vi "increment Modbus address.vi"(0 "available addresses":T1(array[cluster]), 5 "modbus type":T2, 7 "data type":T3) -> (4 "available addresses out":T1(array[cluster]), 6 "starting address":u16, 8 "subindex (bool)":i32)   [LabVIEW 2013, in "Modbus Slave configuration.lvclass"]
uses:
  Modbus Slave configuration.lvclass
  <vilib>/NI/Tag Bus/tag/Data Type.ctl
  <vilib>/NI/Tag Bus/tag/tag descriptor.lvclass
  module channel/data bank type.ctl
  module channel/Modbus Module Channel.lvclass
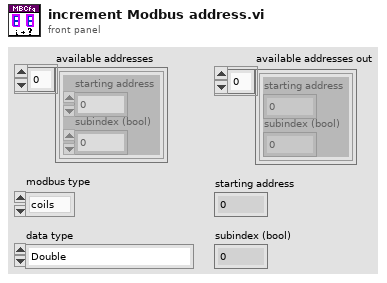
[diagram p1: front panel]
types:
  T1 = cluster{"starting address":u16, "subindex (bool)":i32}[]
  T2 = typedef "Modbus Module Channel.lvclass/data bank type.ctl" = enum16{"coils", "discrete inputs", "input registers", "holding registers"}
  T3 = typedef "tag bus.lvlib/tag descriptor.lvclass/Data Type.ctl" = enum16{"Double", "Single", "I64", "I32", "I16", "I8", "U64", "U32", "U16", "U8", "Boolean", "String", "Array of Double", "Array of Single", "Array of I64", "Array of I32", "Array of I16", "Array of I8", "Array of U64", "Array of U32", "Array of U16", "Array of U8", "Array of Boolean", "Array of String"}
  T4 = cluster{"starting address":u16, "subindex (bool)":i32}
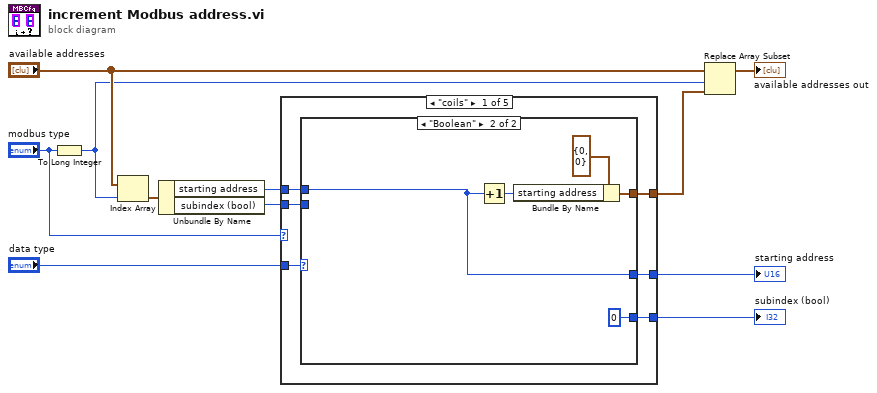
[diagram p0: block diagram]
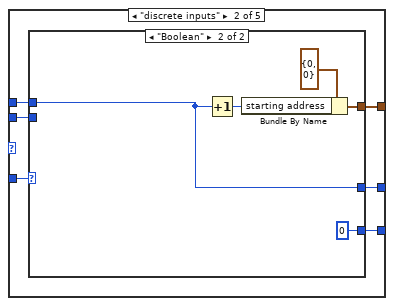
[diagram p3: hidden frame]
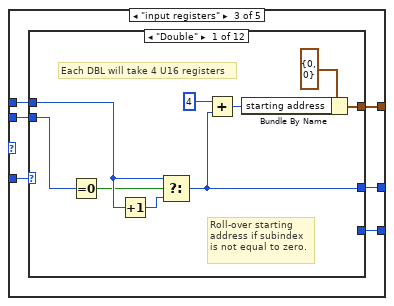
[diagram p5: hidden frame]
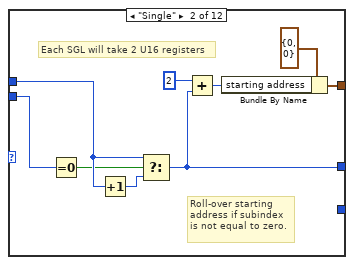
[diagram p6: hidden frame]
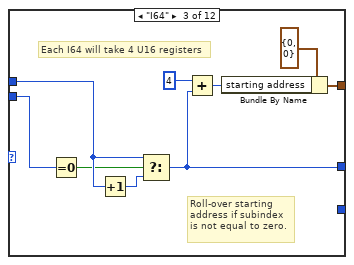
[diagram p7: hidden frame]
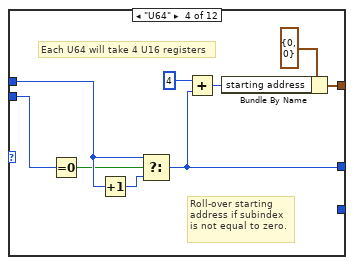
[diagram p8: hidden frame]
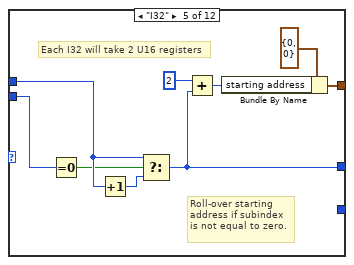
[diagram p9: hidden frame]
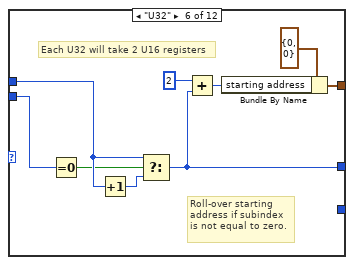
[diagram p10: hidden frame]
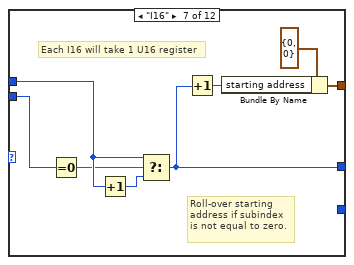
[diagram p11: hidden frame]
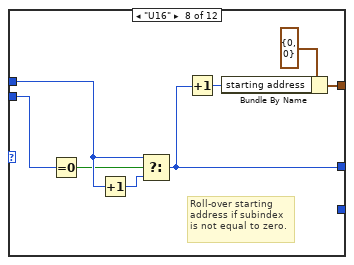
[diagram p12: hidden frame]
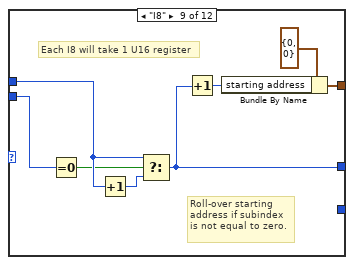
[diagram p13: hidden frame]
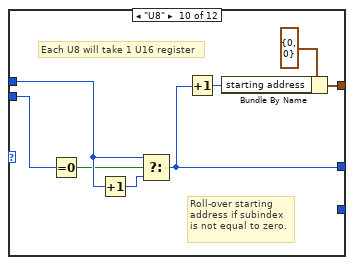
[diagram p14: hidden frame]
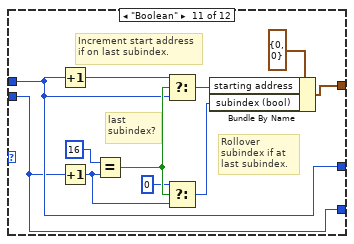
[diagram p15: hidden frame]
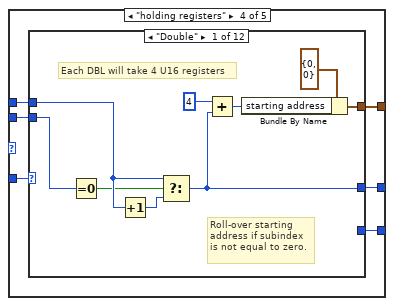
[diagram p17: hidden frame]
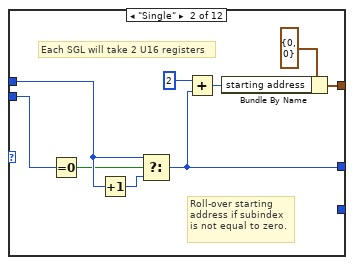
[diagram p18: hidden frame]
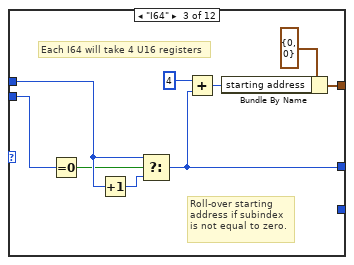
[diagram p19: hidden frame]
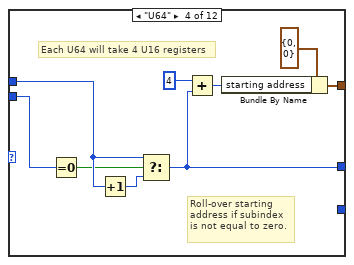
[diagram p20: hidden frame]
diagram:
  n1 = To Long Integer(number="modbus type") -> (32bit integer=w8:i32)
  n2 = Index Array(array="available addresses", index=w8) -> (element=w10:T4)
  n3 = Unbundle By Name(w10) -> ("starting address"=w4:u16, "subindex (bool)"=w7:i32)
  n4 = case shown="\"coils\"" "modbus type" {
    tunnel: "data type" -> [w17 w28 w39 w142 _]
    tunnel: w7 -> [w16 w27 w38 w141 _]
    tunnel: [w15 w26 w37 w140 _] -> w5
    tunnel: w4 -> [w14 w25 w36 w139 _]
    tunnel: [w13 w24 w35 w138 _] -> w3
    tunnel: [w12 w23 w34 w137 _] -> w2
    frame "coils" {
      n5 = case shown="\"Boolean\"" w17 {
        tunnel: w16 -> [_ _]
        tunnel: w14 -> [_ w18]
        tunnel: [_ w21] -> w15
        tunnel: [_ w18] -> w13
        tunnel: [_ 0 ("subindex (bool)")] -> w12
        frame Default {
        }
        frame "Boolean" {
          n6 = Increment(x=w18) -> (x+1=w20:u16)
          n7 = Bundle By Name(cluster=T4 {"starting address"=0, "subindex (bool)"=0} ("element"), "starting address"=w20) -> (w21:T4)
        }
      }
    }
    frame "discrete inputs" {
      n8 = case shown="\"Boolean\"" w28 {
        tunnel: w27 -> [_ _]
        tunnel: w25 -> [_ w29]
        tunnel: [_ w32] -> w26
        tunnel: [_ w29] -> w24
        tunnel: [_ 0 ("subindex (bool)")] -> w23
        frame Default {
        }
        frame "Boolean" {
          n9 = Increment(x=w29) -> (x+1=w31:u16)
          n10 = Bundle By Name(cluster=T4 {"starting address"=0, "subindex (bool)"=0} ("element"), "starting address"=w31) -> (w32:T4)
        }
      }
    }
    frame "input registers" {
      n11 = case shown="\"Double\"" w39 {
        tunnel: w38 -> [w45 w54 w63 w72 w81 w90 w99 w107 w115 w123 w126 _]
        tunnel: w36 -> [w44 w53 w62 w71 w80 w89 w98 w106 w114 w122 w127 _]
        tunnel: [w47 w56 w65 w74 w83 w92 w100 w108 w116 w124 w135 _] -> w37
        tunnel: [w41 w50 w59 w68 w77 w86 w95 w103 w111 w119 w127 _] -> w35
        tunnel: [_ _ _ _ _ _ _ _ _ _ w126 _] -> w34
        frame "Double" {
          # "Each DBL will take 4 U16 registers"
          # "Roll-over starting\naddress if subindex\nis not equal to zero."
          n12 = Equal To 0?(x=w45) -> (x = 0?=w42:bool)
          n13 = Increment(x=w44) -> (x+1=w43:u16)
          n14 = Select(t=w44, s=w42, f=w43) -> (s? t:f=w41:u16)
          n15 = Add(x=u16 4, y=w41) -> (x+y=w40:u16)
          n16 = Bundle By Name(cluster=T4 {"starting address"=0, "subindex (bool)"=0} ("element"), "starting address"=w40) -> (w47:T4)
        }
        frame "Single" {
          # "Each SGL will take 2 U16 registers"
          # "Roll-over starting\naddress if subindex\nis not equal to zero."
          n17 = Equal To 0?(x=w54) -> (x = 0?=w51:bool)
          n18 = Increment(x=w53) -> (x+1=w52:u16)
          n19 = Select(t=w53, s=w51, f=w52) -> (s? t:f=w50:u16)
          n20 = Add(x=u16 2, y=w50) -> (x+y=w49:u16)
          n21 = Bundle By Name(cluster=T4 {"starting address"=0, "subindex (bool)"=0} ("element"), "starting address"=w49) -> (w56:T4)
        }
        frame "I64" {
          # "Each I64 will take 4 U16 registers"
          # "Roll-over starting\naddress if subindex\nis not equal to zero."
          n22 = Equal To 0?(x=w63) -> (x = 0?=w60:bool)
          n23 = Increment(x=w62) -> (x+1=w61:u16)
          n24 = Select(t=w62, s=w60, f=w61) -> (s? t:f=w59:u16)
          n25 = Add(x=u16 4, y=w59) -> (x+y=w58:u16)
          n26 = Bundle By Name(cluster=T4 {"starting address"=0, "subindex (bool)"=0} ("element"), "starting address"=w58) -> (w65:T4)
        }
        frame "U64" {
          # "Each U64 will take 4 U16 registers"
          # "Roll-over starting\naddress if subindex\nis not equal to zero."
          n27 = Equal To 0?(x=w72) -> (x = 0?=w69:bool)
          n28 = Increment(x=w71) -> (x+1=w70:u16)
          n29 = Select(t=w71, s=w69, f=w70) -> (s? t:f=w68:u16)
          n30 = Add(x=u16 4, y=w68) -> (x+y=w67:u16)
          n31 = Bundle By Name(cluster=T4 {"starting address"=0, "subindex (bool)"=0} ("element"), "starting address"=w67) -> (w74:T4)
        }
        frame "I32" {
          # "Each I32 will take 2 U16 registers"
          # "Roll-over starting\naddress if subindex\nis not equal to zero."
          n32 = Equal To 0?(x=w81) -> (x = 0?=w78:bool)
          n33 = Increment(x=w80) -> (x+1=w79:u16)
          n34 = Select(t=w80, s=w78, f=w79) -> (s? t:f=w77:u16)
          n35 = Add(x=u16 2, y=w77) -> (x+y=w76:u16)
          n36 = Bundle By Name(cluster=T4 {"starting address"=0, "subindex (bool)"=0} ("element"), "starting address"=w76) -> (w83:T4)
        }
        frame "U32" {
          # "Each U32 will take 2 U16 registers"
          # "Roll-over starting\naddress if subindex\nis not equal to zero."
          n37 = Equal To 0?(x=w90) -> (x = 0?=w87:bool)
          n38 = Increment(x=w89) -> (x+1=w88:u16)
          n39 = Select(t=w89, s=w87, f=w88) -> (s? t:f=w86:u16)
          n40 = Add(x=u16 2, y=w86) -> (x+y=w85:u16)
          n41 = Bundle By Name(cluster=T4 {"starting address"=0, "subindex (bool)"=0} ("element"), "starting address"=w85) -> (w92:T4)
        }
        frame "I16" {
          # "Each I16 will take 1 U16 register"
          # "Roll-over starting\naddress if subindex\nis not equal to zero."
          n42 = Equal To 0?(x=w99) -> (x = 0?=w96:bool)
          n43 = Increment(x=w98) -> (x+1=w97:u16)
          n44 = Select(t=w98, s=w96, f=w97) -> (s? t:f=w95:u16)
          n45 = Increment(x=w95) -> (x+1=w94:u16)
          n46 = Bundle By Name(cluster=T4 {"starting address"=0, "subindex (bool)"=0} ("element"), "starting address"=w94) -> (w100:T4)
        }
        frame "U16" {
          # "Roll-over starting\naddress if subindex\nis not equal to zero."
          n47 = Equal To 0?(x=w107) -> (x = 0?=w104:bool)
          n48 = Increment(x=w106) -> (x+1=w105:u16)
          n49 = Select(t=w106, s=w104, f=w105) -> (s? t:f=w103:u16)
          n50 = Increment(x=w103) -> (x+1=w102:u16)
          n51 = Bundle By Name(cluster=T4 {"starting address"=0, "subindex (bool)"=0} ("element"), "starting address"=w102) -> (w108:T4)
        }
        frame "I8" {
          # "Each I8 will take 1 U16 register"
          # "Roll-over starting\naddress if subindex\nis not equal to zero."
          n52 = Equal To 0?(x=w115) -> (x = 0?=w112:bool)
          n53 = Increment(x=w114) -> (x+1=w113:u16)
          n54 = Select(t=w114, s=w112, f=w113) -> (s? t:f=w111:u16)
          n55 = Increment(x=w111) -> (x+1=w110:u16)
          n56 = Bundle By Name(cluster=T4 {"starting address"=0, "subindex (bool)"=0} ("element"), "starting address"=w110) -> (w116:T4)
        }
        frame "U8" {
          # "Each U8 will take 1 U16 register"
          # "Roll-over starting\naddress if subindex\nis not equal to zero."
          n57 = Equal To 0?(x=w123) -> (x = 0?=w120:bool)
          n58 = Increment(x=w122) -> (x+1=w121:u16)
          n59 = Select(t=w122, s=w120, f=w121) -> (s? t:f=w119:u16)
          n60 = Increment(x=w119) -> (x+1=w118:u16)
          n61 = Bundle By Name(cluster=T4 {"starting address"=0, "subindex (bool)"=0} ("element"), "starting address"=w118) -> (w124:T4)
        }
        frame "Boolean" {
          # "Increment start address\nif on last subindex."
          # "Rollover subindex if at last subindex."
          # "last\nsubindex?"
          n62 = Increment(x=w127) -> (x+1=w129:u16)
          n63 = Increment(x=w126) -> (x+1=w128:i32)
          n64 = Equal?(x=16, y=w128) -> (x = y?=w133:bool)
          n65 = Select(t=w129, s=w133, f=w127) -> (s? t:f=w131:u16)
          n66 = Select(t=0, s=w133, f=w128) -> (s? t:f=w130:i32)
          n67 = Bundle By Name(cluster=T4 {"starting address"=0, "subindex (bool)"=0} ("element"), "starting address"=w131, "subindex (bool)"=w130) -> (w135:T4)
        }
        frame Default {
        }
      }
    }
    frame "holding registers" {
      n68 = case shown="\"Double\"" w142 {
        tunnel: w141 -> [w148 w157 w166 w175 w184 w193 w202 w210 w218 w226 w229 _]
        tunnel: w139 -> [w147 w156 w165 w174 w183 w192 w201 w209 w217 w225 w230 _]
        tunnel: [w150 w159 w168 w177 w186 w195 w203 w211 w219 w227 w238 _] -> w140
        tunnel: [w144 w153 w162 w171 w180 w189 w198 w206 w214 w222 w230 _] -> w138
        tunnel: [_ _ _ _ _ _ _ _ _ _ w229 _] -> w137
        frame "Double" {
          # "Each DBL will take 4 U16 registers"
          # "Roll-over starting\naddress if subindex\nis not equal to zero."
          n69 = Equal To 0?(x=w148) -> (x = 0?=w145:bool)
          n70 = Increment(x=w147) -> (x+1=w146:u16)
          n71 = Select(t=w147, s=w145, f=w146) -> (s? t:f=w144:u16)
          n72 = Add(x=u16 4, y=w144) -> (x+y=w143:u16)
          n73 = Bundle By Name(cluster=T4 {"starting address"=0, "subindex (bool)"=0} ("element"), "starting address"=w143) -> (w150:T4)
        }
        frame "Single" {
          # "Each SGL will take 2 U16 registers"
          # "Roll-over starting\naddress if subindex\nis not equal to zero."
          n74 = Equal To 0?(x=w157) -> (x = 0?=w154:bool)
          n75 = Increment(x=w156) -> (x+1=w155:u16)
          n76 = Select(t=w156, s=w154, f=w155) -> (s? t:f=w153:u16)
          n77 = Add(x=u16 2, y=w153) -> (x+y=w152:u16)
          n78 = Bundle By Name(cluster=T4 {"starting address"=0, "subindex (bool)"=0} ("element"), "starting address"=w152) -> (w159:T4)
        }
        frame "I64" {
          # "Each I64 will take 4 U16 registers"
          # "Roll-over starting\naddress if subindex\nis not equal to zero."
          n79 = Equal To 0?(x=w166) -> (x = 0?=w163:bool)
          n80 = Increment(x=w165) -> (x+1=w164:u16)
          n81 = Select(t=w165, s=w163, f=w164) -> (s? t:f=w162:u16)
          n82 = Add(x=u16 4, y=w162) -> (x+y=w161:u16)
          n83 = Bundle By Name(cluster=T4 {"starting address"=0, "subindex (bool)"=0} ("element"), "starting address"=w161) -> (w168:T4)
        }
        frame "U64" {
          # "Each U64 will take 4 U16 registers"
          # "Roll-over starting\naddress if subindex\nis not equal to zero."
          n84 = Equal To 0?(x=w175) -> (x = 0?=w172:bool)
          n85 = Increment(x=w174) -> (x+1=w173:u16)
          n86 = Select(t=w174, s=w172, f=w173) -> (s? t:f=w171:u16)
          n87 = Add(x=u16 4, y=w171) -> (x+y=w170:u16)
          n88 = Bundle By Name(cluster=T4 {"starting address"=0, "subindex (bool)"=0} ("element"), "starting address"=w170) -> (w177:T4)
        }
        frame "I32" {
          # "Each I32 will take 2 U16 registers"
          # "Roll-over starting\naddress if subindex\nis not equal to zero."
          n89 = Equal To 0?(x=w184) -> (x = 0?=w181:bool)
          n90 = Increment(x=w183) -> (x+1=w182:u16)
          n91 = Select(t=w183, s=w181, f=w182) -> (s? t:f=w180:u16)
          n92 = Add(x=u16 2, y=w180) -> (x+y=w179:u16)
          n93 = Bundle By Name(cluster=T4 {"starting address"=0, "subindex (bool)"=0} ("element"), "starting address"=w179) -> (w186:T4)
        }
        frame "U32" {
          # "Each U32 will take 2 U16 registers"
          # "Roll-over starting\naddress if subindex\nis not equal to zero."
          n94 = Equal To 0?(x=w193) -> (x = 0?=w190:bool)
          n95 = Increment(x=w192) -> (x+1=w191:u16)
          n96 = Select(t=w192, s=w190, f=w191) -> (s? t:f=w189:u16)
          n97 = Add(x=u16 2, y=w189) -> (x+y=w188:u16)
          n98 = Bundle By Name(cluster=T4 {"starting address"=0, "subindex (bool)"=0} ("element"), "starting address"=w188) -> (w195:T4)
        }
        frame "I16" {
          # "Each I16 will take 1 U16 register"
          # "Roll-over starting\naddress if subindex\nis not equal to zero."
          n99 = Equal To 0?(x=w202) -> (x = 0?=w199:bool)
          n100 = Increment(x=w201) -> (x+1=w200:u16)
          n101 = Select(t=w201, s=w199, f=w200) -> (s? t:f=w198:u16)
          n102 = Increment(x=w198) -> (x+1=w197:u16)
          n103 = Bundle By Name(cluster=T4 {"starting address"=0, "subindex (bool)"=0} ("element"), "starting address"=w197) -> (w203:T4)
        }
        frame "U16" {
          # "Roll-over starting\naddress if subindex\nis not equal to zero."
          n104 = Equal To 0?(x=w210) -> (x = 0?=w207:bool)
          n105 = Increment(x=w209) -> (x+1=w208:u16)
          n106 = Select(t=w209, s=w207, f=w208) -> (s? t:f=w206:u16)
          n107 = Increment(x=w206) -> (x+1=w205:u16)
          n108 = Bundle By Name(cluster=T4 {"starting address"=0, "subindex (bool)"=0} ("element"), "starting address"=w205) -> (w211:T4)
        }
        frame "I8" {
          # "Each I8 will take 1 U16 register"
          # "Roll-over starting\naddress if subindex\nis not equal to zero."
          n109 = Equal To 0?(x=w218) -> (x = 0?=w215:bool)
          n110 = Increment(x=w217) -> (x+1=w216:u16)
          n111 = Select(t=w217, s=w215, f=w216) -> (s? t:f=w214:u16)
          n112 = Increment(x=w214) -> (x+1=w213:u16)
          n113 = Bundle By Name(cluster=T4 {"starting address"=0, "subindex (bool)"=0} ("element"), "starting address"=w213) -> (w219:T4)
        }
        frame "U8" {
          # "Each U8 will take 1 U16 register"
          # "Roll-over starting\naddress if subindex\nis not equal to zero."
          n114 = Equal To 0?(x=w226) -> (x = 0?=w223:bool)
          n115 = Increment(x=w225) -> (x+1=w224:u16)
          n116 = Select(t=w225, s=w223, f=w224) -> (s? t:f=w222:u16)
          n117 = Increment(x=w222) -> (x+1=w221:u16)
          n118 = Bundle By Name(cluster=T4 {"starting address"=0, "subindex (bool)"=0} ("element"), "starting address"=w221) -> (w227:T4)
        }
        frame "Boolean" {
          # "Increment start address\nif on last subindex."
          # "Rollover subindex if at last subindex."
          # "last\nsubindex?"
          n119 = Increment(x=w230) -> (x+1=w232:u16)
          n120 = Increment(x=w229) -> (x+1=w231:i32)
          n121 = Equal?(x=16, y=w231) -> (x = y?=w236:bool)
          n122 = Select(t=w232, s=w236, f=w230) -> (s? t:f=w234:u16)
          n123 = Select(t=0, s=w236, f=w231) -> (s? t:f=w233:i32)
          n124 = Bundle By Name(cluster=T4 {"starting address"=0, "subindex (bool)"=0} ("element"), "starting address"=w234, "subindex (bool)"=w233) -> (w238:T4)
        }
        frame Default {
        }
      }
    }
    frame Default {
    }
  }
  "subindex (bool)" <- w2
  "starting address" <- w3
  n125 = Replace Array Subset(array="available addresses", new element=w5, index=w8) -> (→"available addresses out":T1)
